vi "Title.vi"(11 "Front Panel Window:Title":string="Production Interface") -> (3 "Title":string)   [LabVIEW 2025, in "Full User Interface.lvlib"]
uses:
  Full User Interface.lvlib
  Localization/Section.ctl
  Localization/Localization.lvlib
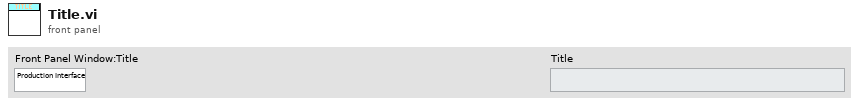
[diagram p1: front panel]
types:
  T1 = typedef "Localization.lvlib/Section.ctl" = enum16{"Menu", "Title", "Workstation Config", "TestInterface"}
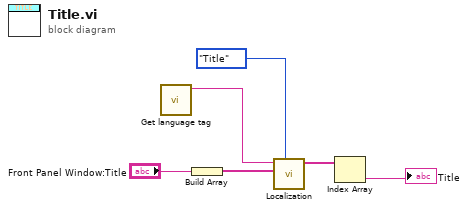
[diagram p0: block diagram]
diagram:
  n1 = call "Get language tag.vi"() -> ("language tag"=w4:string)  [unwired: 11 in]
  n2 = Build Array("Front Panel Window:Title") -> (w5:string[])
  n3 = call "Localization.vi"("section"=Section."Title", "key"=w5, "Language key"=w4) -> ("Value"=w2:string[])  [unwired: 7 in, 1 out]
  n4 = Index Array(array=w2) -> (element=→"Title":string)  [unwired: 1 in]
